vi "Follow 1D Motion Profile.vi"(0 "auton ref":T1={"Starting Pos"=0, "Defence"=enum."Chivel De Fris", "Drivetrain"={"DevStatus"={"status"=FALSE, "code"=0, "source"=""}, "Motors[]"=[], "Square Inputs"=FALSE, "Max Output"=1.0}, "State"=enum."Drive to Outerworks", "Encoder Right"={"DevStatus"={"status"=FALSE, "code"=0, "source"=""}, "EncoderIndex"=enum."Invalid", "CounterIndex"=enum."Invalid", "DistancePerCount"=1.0, "Decoding Type"=enum."4x"}, "Encoder Left"={"DevStatus"={"status"=FALSE, "code"=0, "source"=""}, "EncoderIndex"=enum."Invalid", "CounterIndex"=enum."Invalid", "DistancePerCount"=1.0, "Decoding Type"=enum."4x"}, "Line Sensor"={"DevStatus"={"status"=FALSE, "code"=0, "source"=""}, "DIO Channel"=enum."Invalid", "CntIndex"=enum."Invalid", "Normally Closed"=FALSE}, "navX"={"Interface"={"Protocol"=enum."SERIAL", "Update Rate (4Hz-60Hz)"=4, "navX Open TypeDef"=variant}, "Notify Packet"=refnum, "Loop VI Refnum"=refnum, "Ready to Close Occurrence Refnum"=refnum}, "Front Arm"={"DevStatus"={"status"=FALSE, "code"=0, "source"=""}, "Analog Channel"=enum."Invalid", "Invert Output"=FALSE}, "Start Time"=0, "State Vars"=variant} {"navX"."Interface"."Update Rate (4Hz-60Hz)" min=4 max=60 step=1}, 1 "output range":cluster{"output high":dbl, "output low":dbl}={"output high"=1.0, "output low"=-1.0} {"output low" format="%.2f"; "output high" format="%.2f"}, 2 "Yaw Input? (F)":bool, 3 "Kp_Yaw":dbl, 5 "Profile":T23, 7 "Target Yaw":dbl, 9 "Kv":dbl, 11 "Ka":dbl, 12 "Period (s)":dbl=0.005, 14 "PID gains":T22 {"derivative time (Td, min)" format="%.3f"; "integral time (Ti, min)" format="%.3f"; "proportional gain (Kc)" format="%.3f"}) -> ()   [LabVIEW 2015]
uses:
  Typedef/Motion Profile.ctl
  Typedef/AutonRefType.ctl
  Typedef/Defences.ctl
  <vilib>/Rock Robotics/WPI/RobotDrive/WPI_RobotDriveDevRef.ctl
  <vilib>/Rock Robotics/WPI/MotorControl/WPI_MotorControlDeviceRef.ctl
  <vilib>/Rock Robotics/WPI/MotorControl/WPI_MotorControlType.ctl
  <vilib>/Rock Robotics/SystemInterfaces/DIO/FPGA_DIOPWMChannel.ctl
  <vilib>/Rock Robotics/WPI/PWM/WPI_PWMDeadband.ctl
  <vilib>/Rock Robotics/WPI/CAN/Jaguar/SubVIs/WPI_CANJaguar_ControlMode.ctl
  <vilib>/Rock Robotics/WPI/CAN/TalonSRX/WPI_CANTalonSRX_APIControlMode.ctl
  Typedef/MainStates.ctl
  <vilib>/Rock Robotics/WPI/Encoder/WPI_EncoderDevRef.ctl
  <vilib>/Rock Robotics/SystemInterfaces/Encoder/FPGA_EncoderIdx.ctl
  <vilib>/Rock Robotics/SystemInterfaces/Counter/FPGA_CounterCtrSystemIndex.ctl
  <vilib>/Rock Robotics/WPI/Encoder/WPI_EncoderType.ctl
  <vilib>/Rock Robotics/WPI/Switch/WPI_SwitchDevRef.ctl
  <vilib>/Rock Robotics/SystemInterfaces/DIO/FPGA_DIOChannel.ctl
  NavX/TypeDefs/Z900_navX_DeviceTypeDef.ctl
  NavX/TypeDefs/Z900_navX_ProtocolTypeDef.ctl
  NavX/TypeDefs/Z900_navX_NotifyPacketTypeDef.ctl
  NavX/TypeDefs/Z900_navX_ActionTypeDef.ctl
  <vilib>/Rock Robotics/WPI/Potentiometer/WPI_PotentiometerDevRef.ctl
  <vilib>/Rock Robotics/SystemInterfaces/AI/FPGA_AIChannel.ctl
  <vilib>/Platform/TimedLoop/XDataNode/timing_clust.ctl
  <vilib>/Platform/TimedLoop/XDataNode/nitl_modes.ctl
  <vilib>/Platform/TimedLoop/XDataNode/wakeup.ctl
  <vilib>/addons/control/pid/pid.llb/PID (DBL).vi
  <vilib>/Rock Robotics/WPI/RobotDrive/WPI_RobotDriveArcadeDrive_RatioCurve.vi
  <vilib>/Platform/TimedLoop/XDataNode/XDataNode.xnode
  <vilib>/Platform/TimedLoop/XDataNode/XDNodeRunTimeDep.lvlib
  <vilib>/addons/control/pid/NI_PID_pid.lvlib
  NavX/navX Library v2.lvlib
panel:
  out "Waveform Chart":cluster{dbl, "output":dbl, dbl, dbl, dbl}(graph)
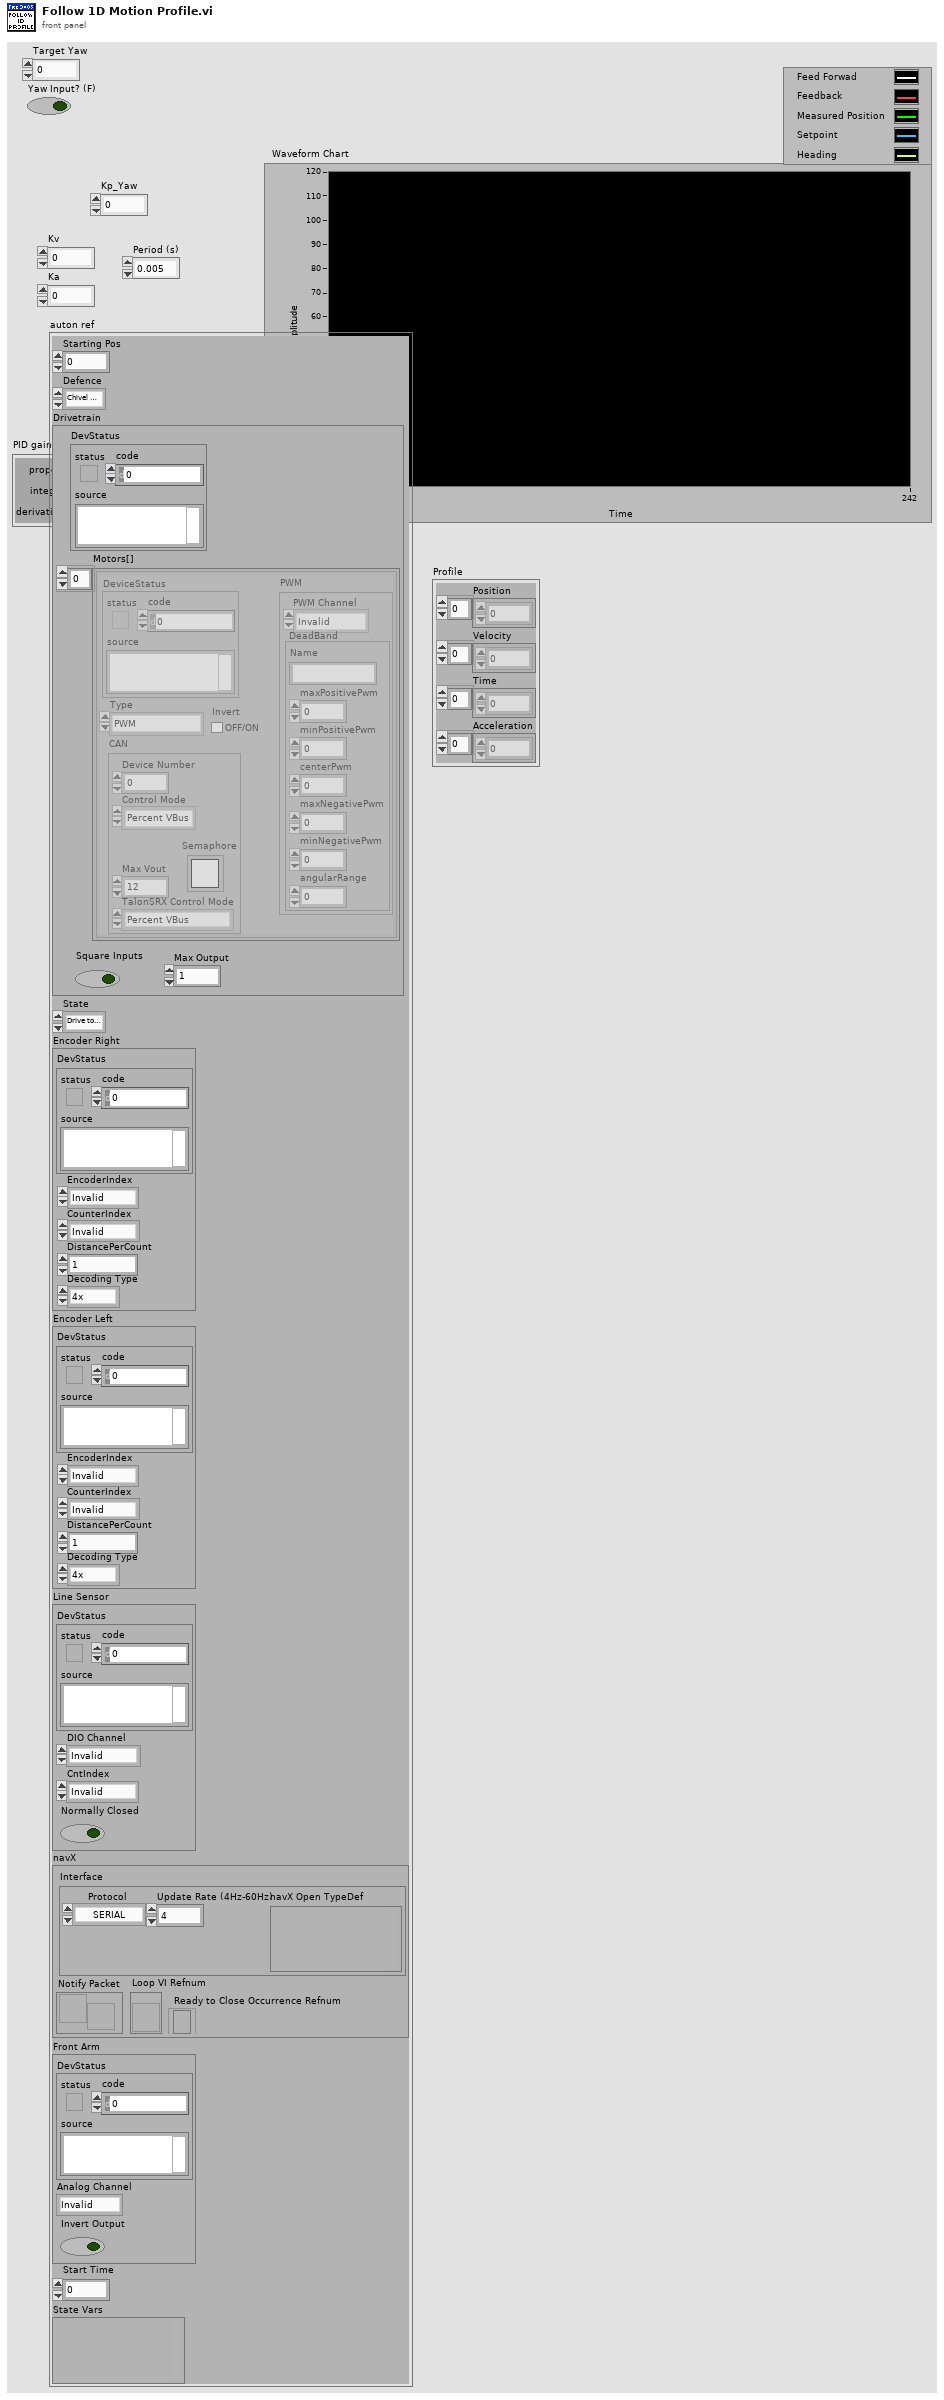
[diagram p1: front panel]
types:
  T1 = typedef "AutonRefType.ctl" = cluster{"Starting Pos":u32, "Defence":T2, "Drivetrain":T3, "State":T11, "Encoder Right":T12, "Encoder Left":T12, "Line Sensor":T16, "navX":T18, "Front Arm":T20, "Start Time":u32, "State Vars":variant}
  T2 = typedef "Defences.ctl" = enum16{"Low Bar", "Chivel De Fris", "Sally Port", "Portcullis", "Draw Bridge", "Moat", "Rough Terrain", "Ramparts", "Rock Wall"}
  T3 = typedef "WPI_RobotDriveDevRef.ctl" = cluster{"DevStatus":errorcluster, "Motors[]":T4[], "Square Inputs":bool, "Max Output":dbl}
  T4 = typedef "WPI_MotorControlDeviceRef.ctl" = cluster{"DeviceStatus":errorcluster, "Type":T5, "PWM":cluster{"PWM Channel":T6, "DeadBand":T7}, "CAN":cluster{"Device Number":u8, "Control Mode":T8, "Semaphore":T9, "Max Vout":dbl, "TalonSRX Control Mode":T10}, "Invert":bool}
  T5 = typedef "WPI_MotorControlType.ctl" = enum16{"PWM", "CAN", "CANTalonSRX"}
  T6 = typedef "FPGA_DIOPWMChannel.ctl" = enum8{"PWM 0", "PWM 1", "PWM 2", "PWM 3", "PWM 4", "PWM 5", "PWM 6", "PWM 7", "PWM 8", "PWM 9", "PWM MXP 0", "PWM MXP 1", "PWM MXP 2", "PWM MXP 3", "PWM MXP 4", "PWM MXP 5", "PWM MXP 6", "PWM MXP 7", "PWM MXP 8", "PWM MXP 9", "Invalid"}
  T7 = typedef "WPI_PWMDeadband.ctl" = cluster{"Name":string, "maxPositivePwm":i32, "minPositivePwm":i32, "centerPwm":i32, "maxNegativePwm":i32, "minNegativePwm":i32, "angularRange":u16}
  T8 = typedef "WPI_CANJaguar_ControlMode.ctl" = enum8{"Percent VBus", "Current", "Speed", "Position", "Voltage"}
  T9 = typedef "Semaphore RefNum" = refnum<k1>
  T10 = typedef "WPI_CANTalonSRX_APIControlMode.ctl" = enum8{"Percent VBus", "Speed", "Position", "Slave", "Unchanged / Invalid", "Voltage Compensation", "Current", "Motion Profile"}
  T11 = typedef "MainStates.ctl" = enum16{"Drive to Outerworks", "Cross Defence", "Align to Line", "Turn to Goal", "Find Position", "Find Distance", "Drive to Scoring Location", "Score Low Goal", "SquareToField", "Hit Driver Station Wall", "Drive Back to Position", "CDF", "Cleanup", "_TEST_Profile", "_TEST_TurnProfile", "_TEST_Impulse", "Error"}
  T12 = typedef "WPI_EncoderDevRef.ctl" = cluster{"DevStatus":errorcluster, "EncoderIndex":T13, "CounterIndex":T14, "DistancePerCount":dbl, "Decoding Type":T15}
  T13 = typedef "FPGA_EncoderIdx.ctl" = enum8{"Enc 0", "Enc 1", "Enc 2", "Enc 3", "Enc 4", "Enc 5", "Enc 6", "Enc 7", "Invalid"}
  T14 = typedef "FPGA_CounterCtrSystemIndex.ctl" = enum8{"Ctr 0", "Ctr 1", "Ctr 2", "Ctr 3", "Ctr 4", "Ctr 5", "Ctr 6", "Ctr 7", "Invalid"}
  T15 = typedef "WPI_EncoderType.ctl" = enum16{"1x", "2x", "4x"}
  T16 = typedef "WPI_SwitchDevRef.ctl" = cluster{"DevStatus":errorcluster, "DIO Channel":T17, "CntIndex":T14, "Normally Closed":bool}
  T17 = typedef "FPGA_DIOChannel.ctl" = enum8{"DIO 0", "DIO 1", "DIO 2", "DIO 3", "DIO 4", "DIO 5", "DIO 6", "DIO 7", "DIO 8", "DIO 9", "DIO MXP 0", "DIO MXP 1", "DIO MXP 2", "DIO MXP 3", "DIO MXP 4", "DIO MXP 5", "DIO MXP 6", "DIO MXP 7", "DIO MXP 8", "DIO MXP 9", "DIO MXP 10", "DIO MXP 11", "DIO MXP 12", "DIO MXP 13", "DIO MXP 14", "DIO MXP 15", "Invalid"}
  T18 = typedef "navX Library v2.lvlib/Z900_navX_DeviceTypeDef.ctl" = cluster{"Interface":cluster{"Protocol":T19, "Update Rate (4Hz-60Hz)":u8, "navX Open TypeDef":variant}, "Notify Packet":refnum<notifier>, "Loop VI Refnum":refnum<vi>, "Ready to Close Occurrence Refnum":refnum<k4>}
  T19 = typedef "navX Library v2.lvlib/Z900_navX_ProtocolTypeDef.ctl" = enum16{"SERIAL", "I2C", "SPI"}
  T20 = typedef "WPI_PotentiometerDevRef.ctl" = cluster{"DevStatus":errorcluster, "Analog Channel":T21, "Invert Output":bool}
  T21 = typedef "FPGA_AIChannel.ctl" = enum8{"AI 0", "AI 1", "AI 2", "AI 3", "AI MXP 0", "AI MXP 1", "AI MXP 2", "AI MXP 3", "Invalid"}
  T22 = cluster{"proportional gain (Kc)":dbl, "integral time (Ti, min)":dbl, "derivative time (Td, min)":dbl}
  T23 = typedef "Motion Profile.ctl" = cluster{"Position":dbl[], "Velocity":dbl[], "Time":dbl[], "Acceleration":dbl[]}
  T24 = cluster{"Yaw":dbl, "Roll":dbl, "Pitch":dbl, "Heading":dbl, "Fused Heading":dbl}
  T25 = typedef "XDNodeRunTimeDep.lvlib/timing_clust.ctl" = cluster{"Expected End [f-1]":u64, "Actual End [f-1]":u64, "Finished Late? [f-1]":bool, "Expected End [i-1]":u64, "Actual End [i-1]":u64, "Finished Late? [i-1]":bool, "Expected Start [i]":u64, "Actual Start [i]":u64, "Expected Start [f]":u64, "Actual Start [f]":u64, "Source Name":string, "Structure Name":string, "Period":i64, "Deadline":i64, "Offset":i64, "Start":i64, "Priority":i32, "Timeout":i32, "Mode":T26, "Wakeup Reason":T27, "Error":errorcluster, "Source Type":string, "Secondary Source Type":string, "Global End Time":u64, "Global Start Time":u64, "Frame Duration":u64, "Iteration Duration":u64, "Assigned CPU":i32, "I/O Scan Engine Mode":u32}
  T26 = typedef "XDNodeRunTimeDep.lvlib/nitl_modes.ctl" = enum32{"No Change", "Process missed periods, maintain original phase", "Discard missed periods, maintain original phase", "Process missed periods, ignore original phase", "Discard missed periods, ignore original phase"}
  T27 = typedef "XDNodeRunTimeDep.lvlib/wakeup.ctl" = enum32{"Normal", "Aborted", "Asynchronous wakeup", "Timing source error", "Timed loop error", "Timeout"}
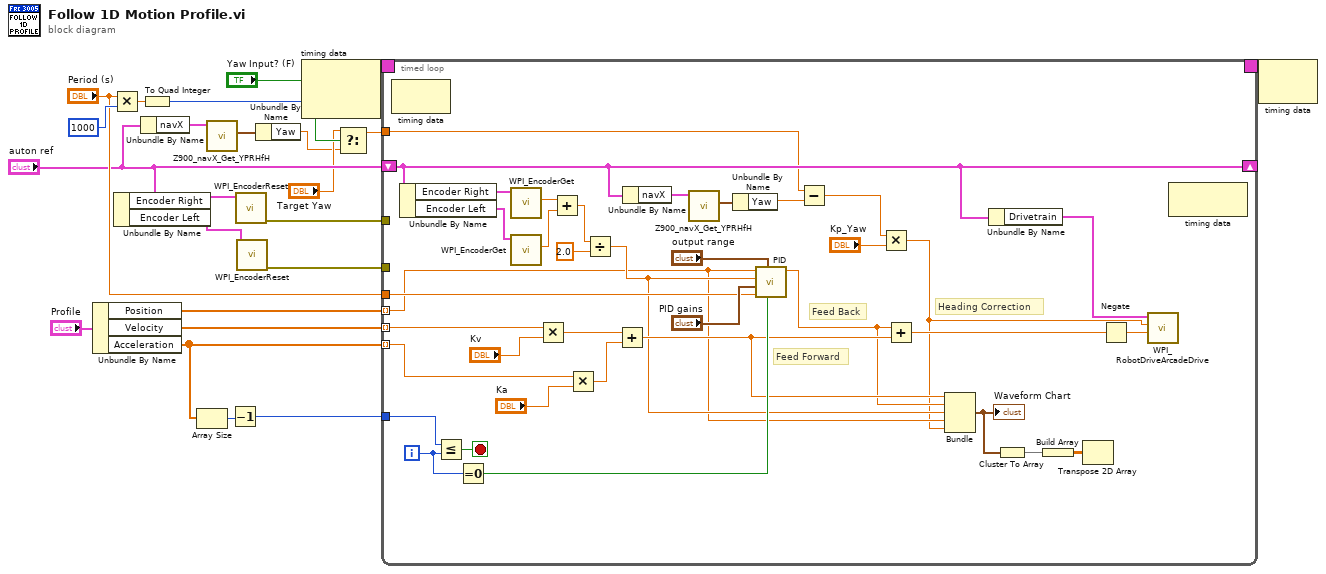
[diagram p0: block diagram]
diagram:
  n1 = Unbundle By Name("Profile") -> ("Position"=w20:dbl[], "Velocity"=w19:dbl[], "Acceleration"=w18:dbl[])
  n2 = Multiply(x="Period (s)", y=1000) -> (x*y=w14:dbl)
  n3 = Unbundle By Name("auton ref") -> ("Encoder Right"=w11:T12, "Encoder Left"=w10:T12)
  n4 = Unbundle By Name("auton ref") -> ("navX"=w7:T18)
  n5 = To Quad Integer(1:w14) -> (0:w13:i64)
  n6 = Array Size(array=w18) -> (size(s)=w17:i32)
  n7 = call "Z900_navX_Get_YPRHfH.vi"("navX Device"=w7) -> ("YRPHfH"=w5:T24)  [unwired: 7 in, 3 out]
  n8 = Decrement(x=w17) -> (x-1=w16:i32)
  n9 = call <vilib>:"WPI_EncoderReset.vi"("EncoderDevRef"=w11) -> ("error out"=w8:errorcluster)  [unwired: 9 in, 1 out]
  n10 = call <vilib>:"WPI_EncoderReset.vi"("EncoderDevRef"=w10) -> ("error out"=w9:errorcluster)  [unwired: 9 in, 1 out]
  n11 = Unbundle By Name(w5) -> ("Yaw"=w1:dbl)
  n12 = node-c288(w13) -> (w23:T25)  [unwired: 1 in]
  n13 = Select(t="Target Yaw", s="Yaw Input? (F)", f=w1) -> (s? t:f=w4:dbl)
  n14 = timed-loop {
    timing: w23 -> [_]
    timing-out: [_] -> w22
    tunnel: w20 -> [w36] mode=indexing
    tunnel: w19 -> [w28] mode=indexing
    tunnel: w18 -> [w43] mode=indexing
    tunnel: w16 -> [w60]
    tunnel: "Period (s)" -> [w52]
    shift-right: [w42] -> _
    shift-left: "auton ref" -> [w42]
    tunnel: w9 -> [_]
    tunnel: w8 -> [_]
    tunnel: w4 -> [w31]
    i -> [w51]
    stop <- w59 stop-if-true
    # "Heading Correction"
    # "Feed Back"
    # "Feed Forward"
    n15 = node-c288() -> ()  [unwired: 1 in, 1 out]
    n16 = Unbundle By Name(w42) -> ("Encoder Right"=w49:T12, "Encoder Left"=w48:T12)
    n17 = Less Or Equal?(x=w60, y=w51) -> (x <= y?=w59:bool)
    n18 = Equal To 0?(x=w51) -> (x = 0?=w50:bool)
    n19 = call <vilib>:"WPI_EncoderGet.vi"("EncoderDevRef"=w49) -> ("Distance"=w47:dbl)  [unwired: 5 in, 5 out]
    n20 = call <vilib>:"WPI_EncoderGet.vi"("EncoderDevRef"=w48) -> ("Distance"=w46:dbl)  [unwired: 5 in, 5 out]
    n21 = Multiply(x=w28, y="Kv") -> (x*y=w56:dbl)
    n22 = Add(x=w47, y=w46) -> (x+y=w45:dbl)
    n23 = Multiply(x=w43, y="Ka") -> (x*y=w55:dbl)
    n24 = Divide(x=w45, y=2.0) -> (x/y=w37:dbl)
    n25 = Add(x=w56, y=w55) -> (x+y=w39:dbl)
    n26 = Unbundle By Name(w42) -> ("navX"=w34:T18)
    n27 = call "Z900_navX_Get_YPRHfH.vi"("navX Device"=w34) -> ("YRPHfH"=w33:T24)  [unwired: 7 in, 3 out]
    n28 = Unbundle By Name(w33) -> ("Yaw"=w32:dbl)
    n29 = call-poly <vilib>:"PID.vi"("reinitialize? (F)"=w50, "output range"="output range", "dt (s)"=w52, "PID gains"="PID gains", "process variable"=w37, "setpoint"=w36) -> ("output"=w38:dbl)  [unwired: 4 in, 1 out]
    n30 = Subtract(x=w31, y=w32) -> (x-y=w30:dbl)
    n31 = Multiply(x=w30, y="Kp_Yaw") -> (x*y=w27:dbl)
    n32 = Add(x=w38, y=w39) -> (x+y=w40:dbl)
    n33 = Bundle(w39, "output"=w38, w37, w36, w27) -> (w26:cluster{dbl, "output":dbl, dbl, dbl, dbl})  [unwired: 1 in]
    "Waveform Chart" <- w26
    n34 = Unbundle By Name(w42) -> ("Drivetrain"=w41:T3)
    n35 = Cluster To Array(cluster=w26) -> (array=w25:dbl[])
    n36 = Build Array(w25) -> (w24:dbl[][])
    n37 = Transpose 2D Array(2D array=w24) -> ()  [unwired: 1 out]
    n38 = Negate(x=w40) -> (-x=w35:dbl)
    n39 = call-poly <vilib>:"WPI_RobotDriveArcadeDrive.vi"("Y axis value (Speed)"=w35, "X axis value (Curve)"=w27, "RobotDriveDevRef"=w41) -> ()  [unwired: 6 in, 3 out]
    n40 = node-c288() -> ()  [unwired: 1 in, 1 out]
  }
  n41 = node-c288(w22) -> ()  [unwired: 1 out]
